vi "myRIO_BRig_RT_dataExp_CueLed.vi"() -> (2 "output_CueLed":i32)   [LabVIEW 2014]
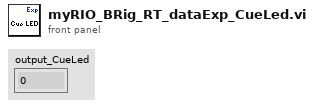
[diagram p1: front panel]
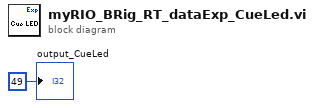
[diagram p0: block diagram]
diagram:
  "output_CueLed" <- 49 ("output_iBlock")
